vi "2.4.vi"() -> ()   [LabVIEW 2011]
uses:
  <vilib>/vision/NI_Vision_Development_Module.lvlib
panel:
  in  "Structuring Element":dbl[][](array[numeric])=[[0.0, 1.0, 0.0], [1.0, 1.0, 1.0], [0.0, 1.0, 0.0]]
  in  "Morphology":u16(ring) items=["(none)", "AutoM", "Close", "Dilate", "Erode", "Gradient", "Open", "Thick", "Thin"]
  in  "Generate":bool
  in  "Look for":enum16{"Bright Objects", "Dark Objects"}(ring)
  in  "Method":T1(ring)=enum."Inter-class Variance"
  out "Binary":T2(plugin-control)
  out "Threshold Range":cluster{"Lower value":sgl, "Upper value":sgl}={"Lower value"=128.0, "Upper value"=255.0} {"Upper value" format="%.2f"; "Lower value" format="%.2f"}
  in  "Stop":bool
  in  "Browse":bool
  out "XY Graph":cluster{dbl[], dbl[]}(graph)
  out "Original Image":T2(plugin-control)
  out "Path to Image":path
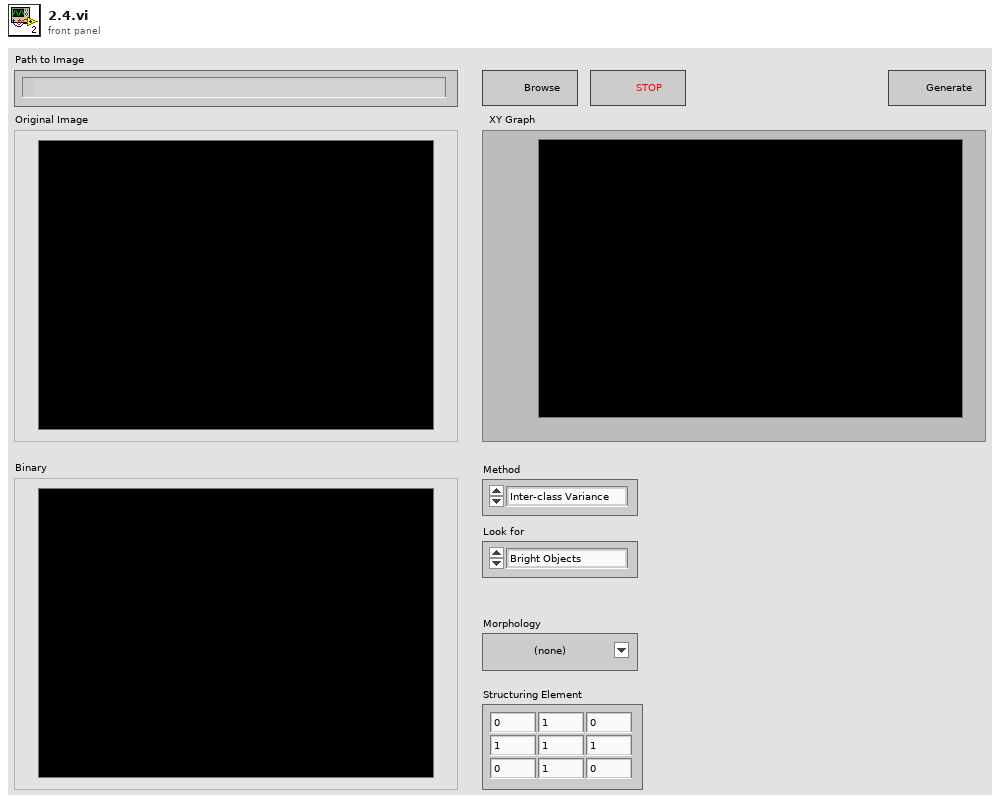
[diagram p1: front panel]
types:
  T1 = enum16{"Clustering", "Entropy", "Metric", "Moments", "Inter-class Variance"}
  T2 = typedef "IMAQ Image.ctl" = refnum<image>
  T3 = typedef "Image Type" = u32
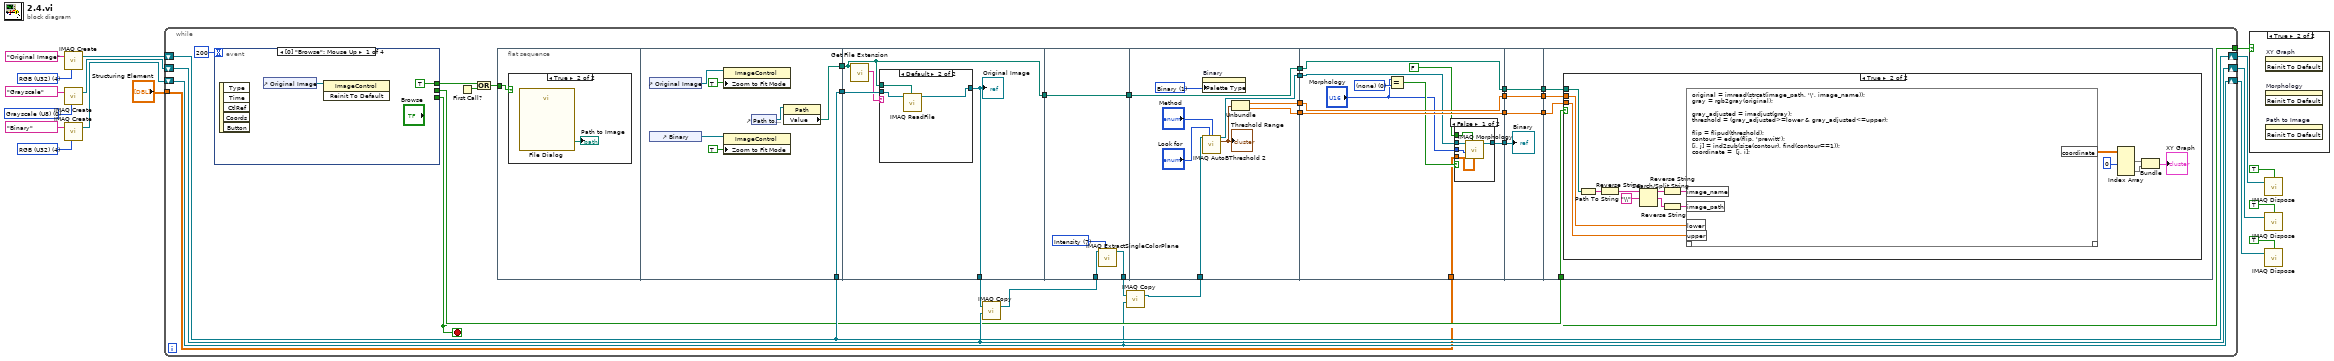
[diagram p0: block diagram]
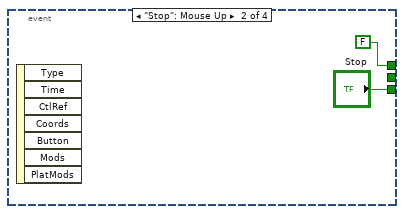
[diagram p3: hidden frame]
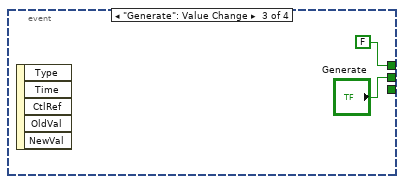
[diagram p4: hidden frame]
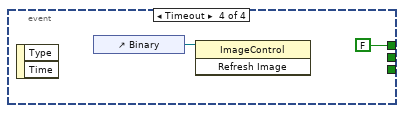
[diagram p5: hidden frame]
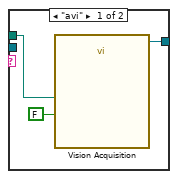
[diagram p7: hidden frame]
diagram:
  w5 = T3 4 items=["Grayscale (U8)", "Grayscale (I16)", "Grayscale (SGL)", "Complex (CSG)", "RGB (U32)", "HSL (U32)", "RGB (U64)", "Grayscale (U16)"] ("Image Type")
  w11 = T3 0 items=["Grayscale (U8)", "Grayscale (I16)", "Grayscale (SGL)", "Complex (CSG)", "RGB (U32)", "HSL (U32)", "RGB (U64)", "Grayscale (U16)"] ("Image Type")
  w16 = T3 4 items=["Grayscale (U8)", "Grayscale (I16)", "Grayscale (SGL)", "Complex (CSG)", "RGB (U32)", "HSL (U32)", "RGB (U64)", "Grayscale (U16)"] ("Image Type")
  n1 = call "IMAQ Create"("Image Name"="Original Image", "Image Type"=w16) -> ("New Image"=w15:T2)  [unwired: 3 in, 1 out]
  n2 = call "IMAQ Create"("Image Name"="Grayscale", "Image Type"=w11) -> ("New Image"=w10:T2)  [unwired: 3 in, 1 out]
  n3 = call "IMAQ Create"("Image Name"="Binary", "Image Type"=w5) -> ("New Image"=w2:T2)  [unwired: 3 in, 1 out]
  n4 = while {
    shift-right: [w41] -> w14
    shift-left: w15 -> [w41]
    tunnel: [w19] -> w13
    shift-right: [w35] -> w8
    shift-left: w10 -> [w35]
    shift-right: [w29] -> w3
    shift-left: w2 -> [w29]
    tunnel: "Structuring Element" -> [w18]
    stop <- w19 stop-if-true
    n5 = event shown="[0] \"Browse\": Mouse Up" {
      selector: _ -> [_ _ _ _]
      dyn-events: _ -> [_ _ _ _]
      timeout: 200 -> [_ _ _ _]
      tunnel: [TRUE FALSE FALSE FALSE] -> w45
      tunnel: [_ "Stop" _ _] -> w19
      tunnel: [_ _ "Generate" _] -> w34
      event "Browse": Mouse Up {
        n6 = event-data() -> ()  [unwired: 1 in, 5 out]
        n7 = control-ref of="Original Image"() -> (w48:refnum<vi>)
        n8 = invoke class="ImageControl" method="Reinit To Default"(reference=w48) -> ()  [unwired: 2 in, 3 out]
      }
      event "Stop": Mouse Up {
        n9 = event-data() -> ()  [unwired: 1 in, 7 out]
      }
      event "Generate": Value Change {
        n10 = event-data() -> ()  [unwired: 1 in, 5 out]
      }
      event Timeout {
        n11 = event-data() -> ()  [unwired: 1 in, 2 out]
        n12 = control-ref of="Binary"() -> (w54:refnum<vi>)
        n13 = invoke class="ImageControl" method="Refresh Image"(reference=w54) -> ()  [unwired: 2 in, 3 out]
      }
    }
    n14 = First Call?() -> (First Call?: T/F=w44:bool)
    n15 = Or(x=w45, y=w44) -> (x .or. y?=w43:bool)
    n16 = flat-sequence {
      tunnel: w43 -> [w55]
      tunnel: [w60] -> w46
      tunnel: [w57] -> w42
      tunnel: w41 -> [w60]
      tunnel: w46 -> [w67]
      tunnel: w42 -> [w64]
      tunnel: [w64] -> w40
      tunnel: [w66] -> w37
      tunnel: w40 -> [w77]
      tunnel: [w77] -> w39
      tunnel: w36 -> [w75]
      tunnel: [w74] -> w30
      tunnel: w39 -> [w86]
      tunnel: [w86] -> w27
      tunnel: [w85] -> w25
      tunnel: [w80] -> w24
      tunnel: [w79] -> w22
      tunnel: w31 -> [w78]
      tunnel: w27 -> [w96]
      tunnel: [w96] -> w26
      tunnel: w25 -> [w93]
      tunnel: w24 -> [w95]
      tunnel: [w95] -> w23
      tunnel: w22 -> [w94]
      tunnel: [w94] -> w21
      tunnel: [w92] -> w20
      tunnel: w18 -> [w87]
      tunnel: w26 -> [w106]
      tunnel: [w106] -> w38
      tunnel: [w105] -> w33
      tunnel: w23 -> [w105]
      tunnel: [w104] -> w32
      tunnel: w21 -> [w104]
      tunnel: w20 -> [w103]
      tunnel: w38 -> [w110]
      tunnel: w34 -> [w109]
      tunnel: w33 -> [w108]
      tunnel: w32 -> [w107]
      frame #0 {
        n17 = case shown="True" w55 {
          frame False {
          }
          frame True {
            n18 = call "File Dialog"() -> ("selected path"=→"Path to Image":path)  [unwired: 12 in, 3 out]
          }
        }
      }
      frame #1 {
        n19 = control-ref of="Original Image"() -> (w63:refnum<vi>)
        n20 = control-ref of="Binary"() -> (w59:refnum<vi>)
        n21 = property class="ImageControl"(reference=w63, "Zoom to Fit Mode"=TRUE) -> ()  [unwired: 1 in, 2 out]
        n22 = property class="ImageControl"(reference=w59, "Zoom to Fit Mode"=TRUE) -> ()  [unwired: 1 in, 2 out]
        n23 = control-ref of="Path to Image"() -> (w61:refnum<vi>)
        n24 = property class="Path"(reference=w61) -> ("Value"=w57:path)  [unwired: 1 in, 2 out]
      }
      frame #2 {
        n25 = call <vilib>:"Get File Extension.vi"("file"=w64) -> ("lowercase file extension"=w65:string)  [unwired: 7 in, 3 out]
        n26 = case shown="Default" w65 {
          tunnel: w67 -> [_ w73]
          tunnel: w64 -> [w70 w72]
          tunnel: [w69 w71] -> w66
          frame "avi" {
            n27 = call "Vision Acquisition"("AVI Path"=w70, "Stop (F)"=FALSE) -> ("Image Out"=w69:T2)  [unwired: 1 in, 24 out]
          }
          frame Default {
            n28 = call "IMAQ ReadFile"("File Path"=w72, "Image"=w73) -> ("Image Out"=w71:T2)  [unwired: 5 in, 4 out]
          }
        }
        "Original Image" <- w66
      }
      frame #3 {
        w76 = 7 items=["Red", "Green", "Blue", "Hue", "Saturation", "Luminance", "Value", "Intensity"] ("Color Plane")
        n29 = call "IMAQ ExtractSingleColorPlane"("Color Plane"=w76, "Image Src"=w75) -> ("Image Dst Out"=w74:T2)  [unwired: 8 in, 1 out]
      }
      frame #4 {
        w84 = u32 1 items=["Grayscale", "Binary", "Gradient", "Rainbow", "Temperature", "User Defined"] ("Palette")
        n30 = property on="Binary" class="ImageControl"("Palette Type"=w84) -> ()  [unwired: 2 in, 2 out]
        n31 = call "IMAQ AutoBThreshold 2"("Image Src"=w78, "Look For (Bright Objects)"="Look for", "Method (clustering)"="Method") -> ("Image Dst Out"=w85:T2, "Threshold Range Out"=w81:cluster{"Lower value":sgl, "Upper value":sgl})  [unwired: 10 in, 1 out]
        "Threshold Range" <- w81
        n32 = Unbundle(w81) -> ("Lower value"=w80:sgl, "Upper value"=w79:sgl)
      }
      frame #5 {
        w90 = u16 0 items=["(none)"]
        n33 = Equal?(x="Morphology", y=w90) -> (x = y?=w89:bool)
        n34 = case shown="False" w89 {
          tunnel: w93 -> [w98 w102]
          tunnel: [w99 w102] -> w92
          tunnel: FALSE -> [w100 _]
          tunnel: "Morphology" -> [w101 _]
          tunnel: w87 -> [w97 _]
          frame False {
            n35 = call "IMAQ Morphology"("Structuring Element"=w97, "Square/Hexa (Square)"=w100, "Operation"=w101, "Image Src"=w98) -> ("Image Dst Out"=w99:T2)  [unwired: 6 in, 1 out]
          }
          frame True {
          }
        }
      }
      frame #6 {
        "Binary" <- w103
      }
      frame #7 {
        n36 = case shown="True" w109 {
          tunnel: w110 -> [_ w125]
          tunnel: w108 -> [_ w112]
          tunnel: w107 -> [_ w111]
          frame False {
          }
          frame True {
            n37 = Path To String(path=w125) -> (string=w124:string)
            n38 = Reverse String(1:w124) -> (0:w123:string)
            n39 = Search/Split String(string=w123, search string/char (-)="\\") -> (substring before match=w121:string, match + rest of string=w120:string)  [unwired: 1 in, 1 out]
            n40 = Reverse String(1:w121) -> (0:w119:string)
            n41 = Reverse String(1:w120) -> (0:w118:string)
            n42 = script code="original = imread(strcat(image_path, '\\', image_name));\ngray = rgb2gray(original);\n\ngray_adjusted = imadjust(gray);\nthreshold = (gray_adjusted>=lower & gray_adjusted<=upper);\n\nflip = flipud(threshold);\ncontour = edge(flip, 'prewitt');\n[i, j] = ind2sub(size(contour), find(contour==1));\ncoordinate =  [j, i];"("image_name"=w119, "image_path"=w118, "lower"=w112, "upper"=w111) -> ("coordinate"=w117:dbl[][])  [unwired: 1 in, 1 out]
            n43 = Index Array(array=w117, index (col) #1=0 ("disabled index (col)")) -> (element #1=w116:dbl[], element #2=w115:dbl[])  [unwired: 3 in]
            n44 = Bundle(w116, w115) -> (→"XY Graph":cluster{dbl[], dbl[]})  [unwired: 1 in]
          }
        }
      }
    }
    n45 = call "IMAQ Copy"("Image Dst"=w35, "Image Src"=w37) -> ("Image Dst Out"=w36:T2)  [unwired: 4 in, 1 out]
    n46 = call "IMAQ Copy"("Image Dst"=w29, "Image Src"=w30) -> ("Image Dst Out"=w31:T2)  [unwired: 4 in, 1 out]
  }
  n47 = case shown="True" w13 {
    frame False {
    }
    frame True {
      n48 = invoke on="XY Graph" class="XYGraph (strict)" method="Reinit To Default"() -> ()  [unwired: 3 in, 3 out]
      n49 = invoke on="Morphology" class="Ring (strict)" method="Reinit To Default"() -> ()  [unwired: 3 in, 3 out]
      n50 = invoke on="Path to Image" class="Path" method="Reinit To Default"() -> ()  [unwired: 3 in, 3 out]
    }
  }
  n51 = call "IMAQ Dispose"("All Images? (No)"=TRUE, "Image"=w14) -> ()  [unwired: 4 in, 1 out]
  n52 = call "IMAQ Dispose"("All Images? (No)"=TRUE, "Image"=w8) -> ()  [unwired: 4 in, 1 out]
  n53 = call "IMAQ Dispose"("All Images? (No)"=TRUE, "Image"=w3) -> ()  [unwired: 4 in, 1 out]
